vi "Begin.vi"() -> (0 "error out":errorcluster)   [LabVIEW 2013]
doc: "Called before other user functions, this VI is expected to open initial I/O refnums, load in file data, and do all program initialization. Notice that the <B>error out</B> terminal is simply used for data flow. Wiring it to other structures or subVIs ensures that this VI runs first."
uses:
  <vilib>/Rock Robotics/WPI/Camera/WPI_CameraImageSize.ctl
  <vilib>/Rock Robotics/SystemInterfaces/DIO/FPGA_DIOPWMChannel.ctl
  <vilib>/Rock Robotics/WPI/DriverStation/WPI_DriverStationRobotMode2.ctl
  <vilib>/Rock Robotics/WPI/Joystick/WPI_JoystickDeviceEnum.ctl
  <vilib>/Rock Robotics/WPI/SafetyOutput/WPI_SafetyOutputConfigMenu.ctl
  <vilib>/Rock Robotics/WPI/Camera/WPI_CameraWhite Balance Values.ctl
  <vilib>/Rock Robotics/WPI/Camera/WPI_CameraExposure Values.ctl
  <vilib>/Rock Robotics/WPI/Camera/WPI_CameraFrameRate.ctl
  <vilib>/Rock Robotics/WPI/RobotDrive/WPI_RobotDriveOpen2MotorWithTalon.vi
  Robot Global Data.vi
  <vilib>/Rock Robotics/WPI/MotorControl/WPI_MotorControlOpen Talon.vi
panel:
  in  "Image Size":T1=enum."160x120"
  out "error out 2":errorcluster
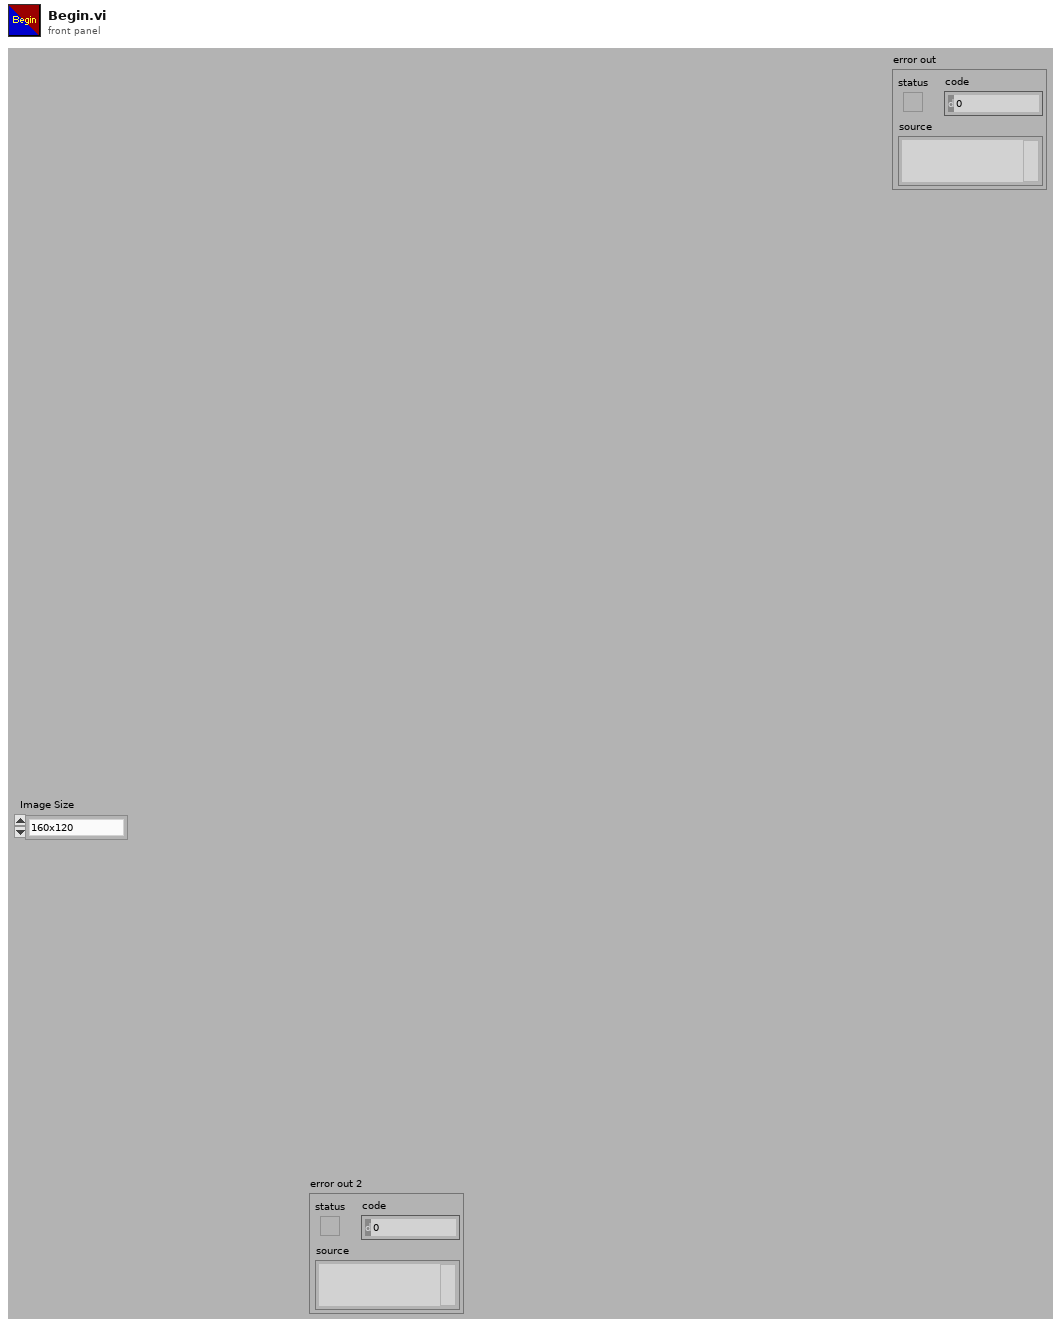
[diagram p1: front panel]
types:
  T1 = typedef "WPI_CameraImageSize.ctl" = enum16{"640x480", "320x240", "160x120"}
  T2 = typedef "WPI_CameraFrameRate.ctl" = u32
  T3 = typedef "WPI_CameraExposure Values.ctl" = enum16{"Auto", "Flicker-free 50 Hz", "Flicker-free 60 Hz", "Hold current"}
  T4 = typedef "WPI_CameraWhite Balance Values.ctl" = enum16{"Auto", "Fixed indoor", "Fixed outdoor 1", "Fixed outdoor 2", "Fixed fluorescent 1", "Fixed fluorescent 2", "Hold current"}
  T5 = typedef "WPI_SafetyOutputConfigMenu.ctl" = enum16{"Enable", "Disable"}
  T6 = typedef "FPGA_DIOPWMChannel.ctl" = enum8{"PWM 1", "PWM 2", "PWM 3", "PWM 4", "PWM 5", "PWM 6", "PWM 7", "PWM 8", "PWM 9", "PWM 10", "Invalid"}
  T7 = typedef "WPI_JoystickDeviceEnum.ctl" = enum16{"USB 1", "USB 2", "USB 3", "USB 4", "Kinect 1", "Kinect 2"}
  T8 = typedef "WPI_DriverStationRobotMode2.ctl" = enum16{"Autonomous Disabled", "Autonomous Enabled", "Teleop Disabled", "Teleop Enabled", "Timeout", "Finish", "Test Disabled", "Test Enabled"}
  T9 = typedef "WPI_CameraDevRef.ctl" = cluster{"Camera Address":string, "CameraStatus":errorcluster, "Acquire Image Notifier":refnum<notifier>}
  T10 = typedef "WPI_RobotDriveDevRef.ctl" = cluster{"DevStatus":errorcluster, "Motors[]":T11[], "Square Inputs":bool, "Max Output":dbl, "Isochronous":bool}
  T11 = typedef "WPI_MotorControlDeviceRef.ctl" = cluster{"DeviceStatus":errorcluster, "Type":enum16{"PWM", "CAN"}, "PWM":cluster{"Digital Module":T12, "PWM Channel":T6, "DeadBand":T13}, "CAN":cluster{"Device Number":u8, "Control Mode":T14, "Semaphore":T15, "Max Vout":dbl}, "Invert":bool, "TransformRef":T16, "InvTransformRef":T16}
  T12 = typedef "FPGA_TypedefDigitalModule.ctl" = enum16{"Digital Module 1", "Digital Module 2"}
  T13 = typedef "WPI_PWMDeadband.ctl" = cluster{"Name":string, "maxPositivePwm":i32, "minPositivePwm":i32, "centerPwm":i32, "maxNegativePwm":i32, "minNegativePwm":i32, "angularRange":u16}
  T14 = typedef "WPI_CANJaguar_ControlMode.ctl" = enum8{"Percent VBus", "Current", "Speed", "Position", "Voltage"}
  T15 = typedef "Semaphore RefNum" = refnum<k1>
  T16 = typedef "WPI_PWMTransform_ConPane.ctl" = refnum<vi>
  T17 = typedef "WPI_JoystickDevRef.ctl" = cluster{"Device":T7}
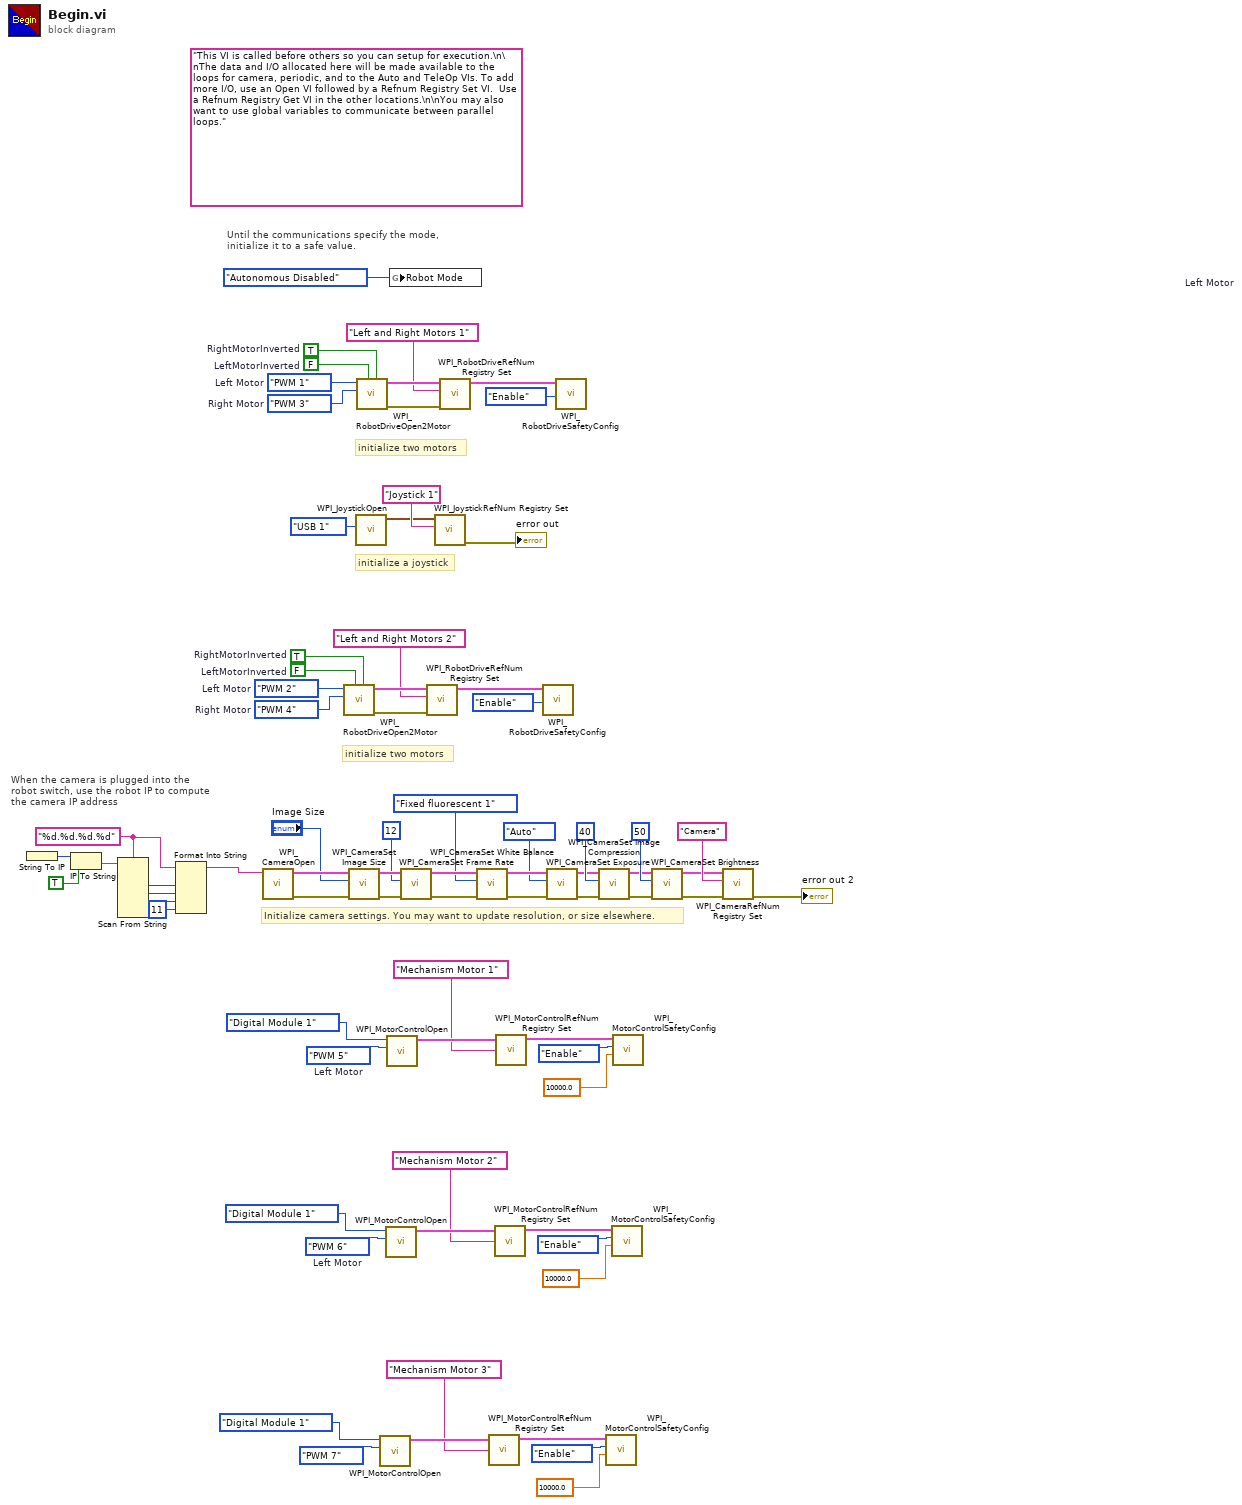
[diagram p0: block diagram]
diagram:
  w4 = "%d.%d.%d.%d" ("format string")
  w38 = FPGA_DIOPWMChannel."PWM 7"  # Left Motor
  w45 = FPGA_DIOPWMChannel."PWM 6"  # Left Motor
  w52 = FPGA_DIOPWMChannel."PWM 5"  # Left Motor
  w55 = FPGA_DIOPWMChannel."PWM 4"  # Right Motor
  w56 = FPGA_DIOPWMChannel."PWM 2"  # Left Motor
  w60 = FALSE  # LeftMotorInverted
  w61 = TRUE  # RightMotorInverted
  (unwired) "This VI is called before others so you can setup for execution.\n\nThe data and I/O allocated here will be made available to the loops for camera, periodic, and to the Auto and TeleOp VIs. To add more I/O, use an Open VI followed by a Refnum Registry Set VI.  Use a Refnum Registry Get VI in the other locations.\n\nYou may also want to use global variables to communicate between parallel loops."
  w69 = FPGA_DIOPWMChannel."PWM 3"  # Right Motor
  w70 = FPGA_DIOPWMChannel."PWM 1"  # Left Motor
  w74 = FALSE  # LeftMotorInverted
  w75 = TRUE  # RightMotorInverted
  # "When the camera is plugged into the\nrobot switch, use the robot IP to compute\nthe camera IP address"
  # "Initialize camera settings. You may want to update resolution, or size elsewhere."
  # "initialize two motors"
  # "initialize a joystick"
  # "Until the communications specify the mode,\ninitialize it to a safe value."
  # "initialize two motors"
  n1 = String To IP() -> (0:w10:u32)  [unwired: 1 in]
  n2 = IP To String(1:TRUE ("dot notation? (F)"), 2:w10) -> (0:w8:string)
  n3 = Scan From String(format string=w4, input string=w8) -> (output 1=w7:i32, output 2=w6:i32, output 3=w5:i32)  [unwired: 7 in, 3 out]
  n4 = Format Into String(format string=w4, w7, w6, w5, 11 ("input 4")) -> (resulting string=w3:string)  [unwired: 2 in, 1 out]
  n5 = call <vilib>:"WPI_CameraOpen.vi"("Camera Address"=w3) -> ("error out"=w22:errorcluster, "CameraDevRef"=w23:T9)  [unwired: 1 in, 8 out]
  n6 = call-poly <vilib>:"WPI_RobotDriveOpen2Motor.vi"("Right Motor Inverted"=w61, "Left Motor Inverted"=w60, "Right Motor"=w55, "Left Motor"=w56) -> ("error out"=w57:errorcluster, "RobotDriveDevRef"=w59:T10)  [unwired: 1 in, 5 out]
  n7 = call <vilib>:"WPI_CameraSet Image Size.vi"("error in (no error)"=w22, "Image Size"="Image Size", "CameraDevRef"=w23) -> ("error out"=w21:errorcluster, "CameraDevRef Out"=w24:T9)  [unwired: 7 out]
  n8 = call <vilib>:"WPI_JoystickOpen.vi"("JoystickDevice"=WPI_JoystickDeviceEnum."USB 1") -> ("JoystickDevRef"=w64:T17)  [unwired: 10 in]
  n9 = call-poly <vilib>:"WPI_RobotDriveOpen2Motor.vi"("Right Motor Inverted"=w75, "Left Motor Inverted"=w74, "Right Motor"=w69, "Left Motor"=w70) -> ("error out"=w71:errorcluster, "RobotDriveDevRef"=w73:T10)  [unwired: 1 in, 5 out]
  n10 = call-poly <vilib>:"WPI_MotorControlOpen.vi"("PWM Channel"=w38, "Digital Module (Module 1)"=enum16{"Digital Module 1"}."Digital Module 1") -> ("MotorControlDeviceRef"=w36:T11)  [unwired: 8 in, 1 out]
  n11 = call-poly <vilib>:"WPI_MotorControlOpen.vi"("PWM Channel"=w45, "Digital Module (Module 1)"=enum16{"Digital Module 1"}."Digital Module 1") -> ("MotorControlDeviceRef"=w43:T11)  [unwired: 8 in, 1 out]
  n12 = call-poly <vilib>:"WPI_MotorControlOpen.vi"("PWM Channel"=w52, "Digital Module (Module 1)"=enum16{"Digital Module 1"}."Digital Module 1") -> ("MotorControlDeviceRef"=w50:T11)  [unwired: 8 in, 1 out]
  n13 = global write "Robot Global Data.vi" "Robot Mode"(WPI_DriverStationRobotMode2."Autonomous Disabled" ("Robot Mode")) -> ()
  n14 = call <vilib>:"WPI_CameraSet Frame Rate.vi"("error in (no error)"=w21, "Frame Rate (fps)"=T2 12, "CameraDevRef"=w24) -> ("error out"=w20:errorcluster, "CameraDevRef Out"=w26:T9)  [unwired: 7 out]
  n15 = call <vilib>:"WPI_RobotDriveRefNum Registry Set.vi"("error in (no error)"=w57, "refnum name"="Left and Right Motors 2", "RobotDriveDevRef"=w59) -> ("RobotDriveDevRef"=w54:T10)  [unwired: 8 out]
  n16 = call <vilib>:"WPI_JoystickRefNum Registry Set.vi"("refnum name"="Joystick 1", "JoystickDevRef"=w64) -> ("error out"=→"error out":errorcluster)  [unwired: 8 in, 1 out]
  n17 = call <vilib>:"WPI_RobotDriveRefNum Registry Set.vi"("error in (no error)"=w71, "refnum name"="Left and Right Motors 1", "RobotDriveDevRef"=w73) -> ("RobotDriveDevRef"=w68:T10)  [unwired: 8 out]
  n18 = call <vilib>:"WPI_CameraSet White Balance.vi"("error in (no error)"=w20, "White Balance"=WPI_CameraWhite_Balance_Values."Fixed fluorescent 1", "CameraDevRef"=w26) -> ("error out"=w19:errorcluster, "CameraDevRef Out"=w25:T9)  [unwired: 7 out]
  n19 = call <vilib>:"WPI_MotorControlRefNum Registry Set.vi"("refnum name"="Mechanism Motor 3", "MotorControlDevRef"=w36) -> ("MotorControlDevRef"=w34:T11)  [unwired: 8 in, 1 out]
  n20 = call <vilib>:"WPI_MotorControlRefNum Registry Set.vi"("refnum name"="Mechanism Motor 2", "MotorControlDevRef"=w43) -> ("MotorControlDevRef"=w41:T11)  [unwired: 8 in, 1 out]
  n21 = call <vilib>:"WPI_MotorControlRefNum Registry Set.vi"("refnum name"="Mechanism Motor 1", "MotorControlDevRef"=w50) -> ("MotorControlDevRef"=w48:T11)  [unwired: 8 in, 1 out]
  n22 = call <vilib>:"WPI_RobotDriveSafetyConfig.vi"("mode"=WPI_SafetyOutputConfigMenu."Enable", "RobotDriveDevRef"=w54) -> ()  [unwired: 8 in, 2 out]
  n23 = call <vilib>:"WPI_CameraSet Exposure.vi"("error in (no error)"=w19, "Exposure"=WPI_CameraExposure_Values."Auto", "CameraDevRef"=w25) -> ("error out"=w18:errorcluster, "CameraDevRef Out"=w28:T9)  [unwired: 7 out]
  n24 = call <vilib>:"WPI_RobotDriveSafetyConfig.vi"("mode"=WPI_SafetyOutputConfigMenu."Enable", "RobotDriveDevRef"=w68) -> ()  [unwired: 8 in, 2 out]
  n25 = call <vilib>:"WPI_CameraSet Image Compression.vi"("error in (no error)"=w18, "Compression"=40, "CameraDevRef"=w28) -> ("error out"=w17:errorcluster, "CameraDevRef Out"=w27:T9)  [unwired: 7 out]
  n26 = call <vilib>:"WPI_MotorControlSafetyConfig.vi"("timeout (s)"=10000.0, "mode"=WPI_SafetyOutputConfigMenu."Enable", "MotorControlDevRef"=w34) -> ()  [unwired: 7 in, 2 out]
  n27 = call <vilib>:"WPI_MotorControlSafetyConfig.vi"("timeout (s)"=10000.0, "mode"=WPI_SafetyOutputConfigMenu."Enable", "MotorControlDevRef"=w41) -> ()  [unwired: 7 in, 2 out]
  n28 = call <vilib>:"WPI_MotorControlSafetyConfig.vi"("timeout (s)"=10000.0, "mode"=WPI_SafetyOutputConfigMenu."Enable", "MotorControlDevRef"=w48) -> ()  [unwired: 7 in, 2 out]
  n29 = call <vilib>:"WPI_CameraSet Brightness.vi"("error in (no error)"=w17, "Brightness"=50, "CameraDevRef"=w27) -> ("error out"=w15:errorcluster, "CameraDevRef Out"=w16:T9)  [unwired: 7 out]
  n30 = call <vilib>:"WPI_CameraRefNum Registry Set.vi"("error in (no error)"=w15, "refnum name"="Camera", "CameraDevRef"=w16) -> ("error out"=→"error out 2":errorcluster)  [unwired: 8 out]
